vi "Get_Encoder.vi"(11 "EncoderDevRef":T1={"DevStatus"={"status"=FALSE, "code"=0, "source"=""}, "EncoderIndex"=enum."Invalid", "CounterIndex"=enum."Invalid", "DistancePerCount"=1.0, "Decoding Type"=enum."4x"}) -> (0 "Encoder Alarm Status":string, 1 "Encoder Direction":string, 2 "Encoder Distance":dbl, 3 "EncoderDevRef 2":T1={"DevStatus"={"status"=FALSE, "code"=0, "source"=""}, "EncoderIndex"=enum."Invalid", "CounterIndex"=enum."Ctr 1", "DistancePerCount"=2.0, "Decoding Type"=enum."4x"})   [LabVIEW 2013]
uses:
  <vilib>/Rock Robotics/WPI/Encoder/WPI_EncoderDevRef.ctl
  <vilib>/Rock Robotics/SystemInterfaces/Encoder/FPGA_EncoderIdx.ctl
  <vilib>/Rock Robotics/SystemInterfaces/Counter/FPGA_CounterCtrSystemIndex.ctl
  <vilib>/Rock Robotics/WPI/Encoder/WPI_EncoderType.ctl
panel:
  out "Encoder Rate (distance/sec)":dbl
  in  "Reset Encoder?":bool
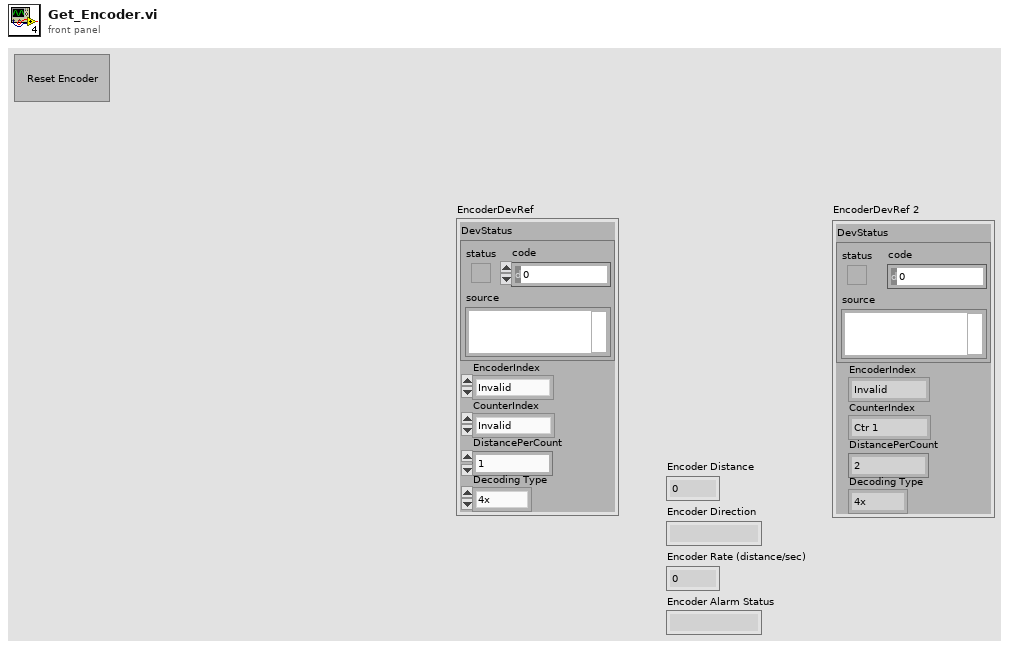
[diagram p1: front panel]
types:
  T1 = typedef "WPI_EncoderDevRef.ctl" = cluster{"DevStatus":errorcluster, "EncoderIndex":T2, "CounterIndex":T3, "DistancePerCount":dbl, "Decoding Type":T4}
  T2 = typedef "FPGA_EncoderIdx.ctl" = enum8{"Enc 0", "Enc 1", "Enc 2", "Enc 3", "Invalid"}
  T3 = typedef "FPGA_CounterCtrSystemIndex.ctl" = enum8{"Ctr 0", "Ctr 1", "Ctr 2", "Ctr 3", "Ctr 4", "Ctr 5", "Ctr 6", "Ctr 7", "Invalid"}
  T4 = typedef "WPI_EncoderType.ctl" = enum16{"1x", "2x", "4x"}
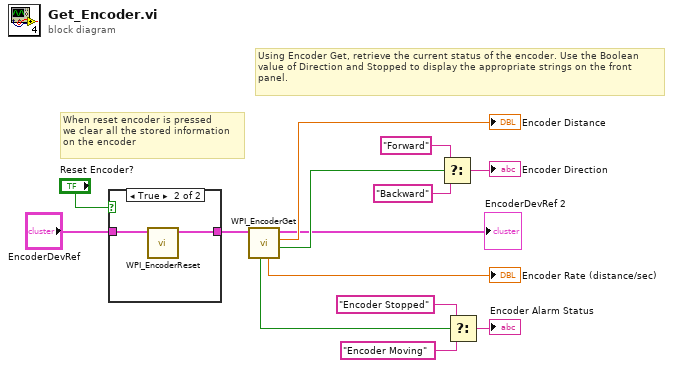
[diagram p0: block diagram]
diagram:
  # "Using Encoder Get, retrieve the current status of the encoder. Use the Boolean value of Direction and Stopped to display the appropriate strings on the front panel."
  # "When reset encoder is pressed\nwe clear all the stored information\non the encoder"
  n1 = case shown="True" "Reset Encoder?" {
    tunnel: "EncoderDevRef" -> [w15 w17]
    tunnel: [w15 w16] -> w12
    frame False {
    }
    frame True {
      n2 = call <vilib>:"WPI_EncoderReset.vi"("EncoderDevRef"=w17) -> ("EncoderDevRef"=w16:T1)  [unwired: 1 in, 9 out]
    }
  }
  n3 = call <vilib>:"WPI_EncoderGet.vi"("EncoderDevRef"=w12) -> ("Direction"=w11:bool, "Distance"=→"Encoder Distance":dbl, "EncoderDevRef"=→"EncoderDevRef 2":T1, "Rate"=→"Encoder Rate (distance/sec)":dbl, "Stopped"=w10:bool)  [unwired: 1 in, 5 out]
  n4 = Select(t="Forward", s=w11, f="Backward") -> (s? t:f=→"Encoder Direction":string)
  n5 = Select(t="Encoder Stopped", s=w10, f="Encoder Moving") -> (s? t:f=→"Encoder Alarm Status":string)
